vi "To String.vi"(8 "error in (no error)":errorcluster, 11 "NT Scalar (Numeric) in":refnum<class "NT Scalar (Numeric).lvclass">) -> (0 "error out":errorcluster, 2 "string":string, 3 "NT Scalar (Numeric) out":refnum<class "NT Scalar (Numeric).lvclass">)   [LabVIEW 2020, in "PV Access.lvlib" / "PV Data.lvlib" / "NT Scalar (Numeric).lvclass"]
uses:
  NT Scalar (Numeric).lvclass
  C:/Users/eyw68381/source/repos/pvaccess-labview/labview/source/PV Data/NT Scalar/NT Scalar.lvclass
  NT Scalar/NT Scalar.lvclass
  NT Scalar (Numeric).lvclass/NT Scalar (Numeric).ctl
  29362789-3a72-4e85-84c0-103a89d78b8d.vi
  70fe9844-d617-4775-a71c-bfed16de9d89.vi
  a1b93c76-8069-4554-a213-bfd5ad968426.vi
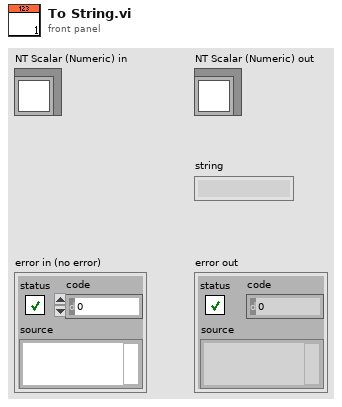
[diagram p1: front panel]
types:
  T1 = typedef "PV Access.lvlib/PV Data.lvlib/Type Code.ctl" = enum8{"Null", "Bool", "BoolA", "Int8", "Int8A", "Int16", "Int16A", "Int32", "Int32A", "Int64", "Int64A", "UInt8", "UInt8A", "UInt16", "UInt16A", "UInt32", "UInt32A", "UInt64", "UInt64A", "Float32", "Float32A", "Float64", "Float64A", "String", "StringA", "Struct", "StructA", "Union", "UnionA", "Any", "AnyA"}
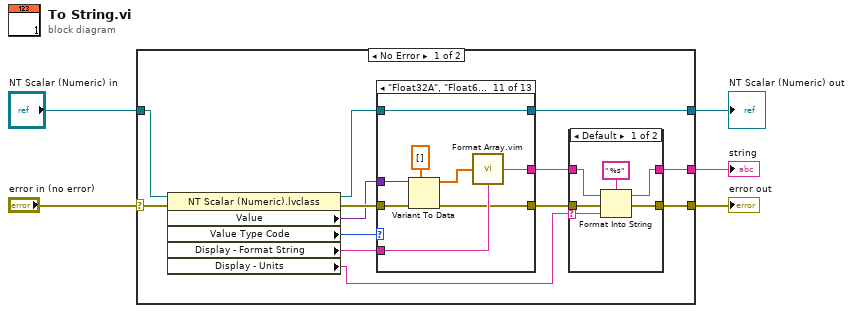
[diagram p0: block diagram]
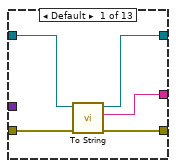
[diagram p3: hidden frame]
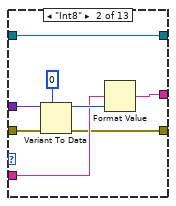
[diagram p4: hidden frame]
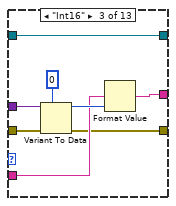
[diagram p5: hidden frame]
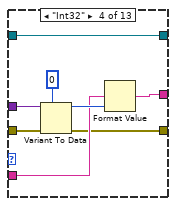
[diagram p6: hidden frame]
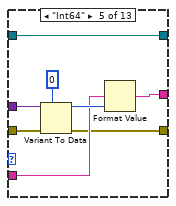
[diagram p7: hidden frame]
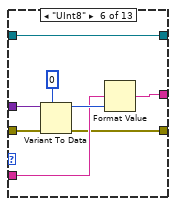
[diagram p8: hidden frame]
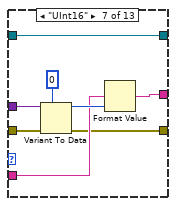
[diagram p9: hidden frame]
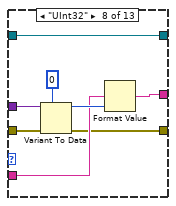
[diagram p10: hidden frame]
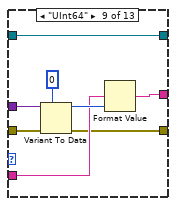
[diagram p11: hidden frame]
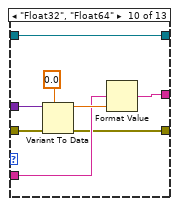
[diagram p12: hidden frame]
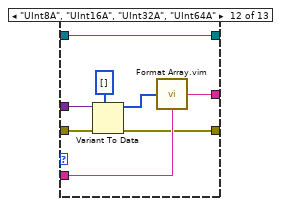
[diagram p13: hidden frame]
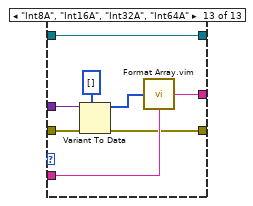
[diagram p14: hidden frame]
diagram:
  n1 = case shown="No Error" "error in (no error)" {
    selector: "error in (no error)" -> [w15 w129]
    tunnel: [w6 w129] -> w2
    tunnel: [w11 w128] -> w1
    tunnel: "NT Scalar (Numeric) in" -> [w14 w128]
    tunnel: [w9 _] -> w3
    frame No Error {
      n2 = property class="NT Scalar (Numeric).lvclass"(reference=w14, error in=w15) -> (reference out=w12:refnum<class "NT Scalar (Numeric).lvclass">, error out=w18:errorcluster, "Value"=w16:variant, "Value Type Code"=w17:T1, "Display - Format String"=w13:string, "Display - Units"=w10:string)
      n3 = case shown="\"Float32A\", \"Float64A\"" w17 {
        tunnel: w18 -> [w31 w37 w45 w53 w61 w69 w77 w85 w93 w101 w110 w118 w126]
        tunnel: w16 -> [_ w38 w46 w54 w62 w70 w78 w86 w94 w102 w111 w119 w127]
        tunnel: [w28 w32 w40 w48 w56 w64 w72 w80 w88 w96 w104 w112 w120] -> w7
        tunnel: [w27 w33 w41 w49 w57 w65 w73 w81 w89 w97 w105 w113 w123] -> w8
        tunnel: w13 -> [_ w34 w42 w50 w58 w66 w74 w82 w90 w98 w106 w114 w122]
        tunnel: w12 -> [w30 w36 w44 w52 w60 w68 w76 w84 w92 w100 w108 w116 w124]
        tunnel: [w29 w36 w44 w52 w60 w68 w76 w84 w92 w100 w108 w116 w124] -> w11
        frame Default {
          n4 = call-parent "To String.vi"("error in (no error)"=w31, "NT Scalar in"=w30) -> ("error out"=w28:errorcluster, "string"=w27:string, "NT Scalar out"=w29:refnum<class "NT Scalar (Numeric).lvclass">)  [unwired: 7 in]
        }
        frame "Int8" {
          n5 = Variant To Data(error in=w37, type=i8 0, Variant=w38) -> (data=w35:i8, error out=w32:errorcluster)
          n6 = Format Value(format string=w34, value (0)=w35) -> (output string=w33:string)  [unwired: 1 in]
        }
        frame "Int16" {
          n7 = Variant To Data(error in=w45, type=i16 0, Variant=w46) -> (data=w43:i16, error out=w40:errorcluster)
          n8 = Format Value(format string=w42, value (0)=w43) -> (output string=w41:string)  [unwired: 1 in]
        }
        frame "Int32" {
          n9 = Variant To Data(error in=w53, type=0, Variant=w54) -> (data=w51:i32, error out=w48:errorcluster)
          n10 = Format Value(format string=w50, value (0)=w51) -> (output string=w49:string)  [unwired: 1 in]
        }
        frame "Int64" {
          n11 = Variant To Data(error in=w61, type=i64 0, Variant=w62) -> (data=w59:i64, error out=w56:errorcluster)
          n12 = Format Value(format string=w58, value (0)=w59) -> (output string=w57:string)  [unwired: 1 in]
        }
        frame "UInt8" {
          n13 = Variant To Data(error in=w69, type=u8 0, Variant=w70) -> (data=w67:u8, error out=w64:errorcluster)
          n14 = Format Value(format string=w66, value (0)=w67) -> (output string=w65:string)  [unwired: 1 in]
        }
        frame "UInt16" {
          n15 = Variant To Data(error in=w77, type=u16 0, Variant=w78) -> (data=w75:u16, error out=w72:errorcluster)
          n16 = Format Value(format string=w74, value (0)=w75) -> (output string=w73:string)  [unwired: 1 in]
        }
        frame "UInt32" {
          n17 = Variant To Data(error in=w85, type=u32 0, Variant=w86) -> (data=w83:u32, error out=w80:errorcluster)
          n18 = Format Value(format string=w82, value (0)=w83) -> (output string=w81:string)  [unwired: 1 in]
        }
        frame "UInt64" {
          n19 = Variant To Data(error in=w93, type=u64 0, Variant=w94) -> (data=w91:u64, error out=w88:errorcluster)
          n20 = Format Value(format string=w90, value (0)=w91) -> (output string=w89:string)  [unwired: 1 in]
        }
        frame "Float32", "Float64" {
          n21 = Variant To Data(error in=w101, type=0.0, Variant=w102) -> (data=w99:dbl, error out=w96:errorcluster)
          n22 = Format Value(format string=w98, value (0)=w99) -> (output string=w97:string)  [unwired: 1 in]
        }
        frame "Float32A", "Float64A" {
          n23 = Variant To Data(error in=w110, type=dbl[] [], Variant=w111) -> (data=w107:dbl[], error out=w104:errorcluster)
          n24 = call "Format Array.vim"("format string"=w106, "array"=w107) -> ("string"=w105:string)  [unwired: 2 in]
        }
        frame "UInt8A", "UInt16A", "UInt32A", "UInt64A" {
          n25 = Variant To Data(error in=w118, type=u64[] [], Variant=w119) -> (data=w115:u64[], error out=w112:errorcluster)
          n26 = call "Format Array.vim"("format string"=w114, "array"=w115) -> ("string"=w113:string)  [unwired: 2 in]
        }
        frame "Int8A", "Int16A", "Int32A", "Int64A" {
          n27 = Variant To Data(error in=w126, type=i64[] [], Variant=w127) -> (data=w121:i64[], error out=w120:errorcluster)
          n28 = call "Format Array.vim"("format string"=w122, "array"=w121) -> ("string"=w123:string)  [unwired: 2 in]
        }
      }
      n29 = case shown="Default" w10 {
        selector: w10 -> [w20 _]
        tunnel: w8 -> [w21 w26]
        tunnel: [w19 w26] -> w9
        tunnel: w7 -> [w23 w25]
        tunnel: [w22 w25] -> w6
        frame Default {
          n30 = Format Into String(format string=" %s", initial string=w21, error in=w23, w20) -> (resulting string=w19:string, error out=w22:errorcluster)
        }
        frame "" {
        }
      }
    }
    frame Error {
    }
  }
  "error out" <- w2
  "NT Scalar (Numeric) out" <- w1
  "string" <- w3
